vi "DIMPowerSupply.constructor.vi"(0 "name":string, 2 "data in":string, 5 "error in (no error)":errorcluster) -> (14 "i ref out":refnum<vi>, 16 "data out":string, 19 "error out":errorcluster)   [LabVIEW 2014, in "DIMPowerSupply.lvlib"]
doc: "This is the constructor of the DIMPowerSupply class.\n\nauthor: Frank Herfurth, CERN\nmaintainer: Frank Herfurth and Dietrich Beck, GSI\n\nLicense Agreement for this software:\n\nCopyright (C)\nGesellschaft für Schwerionenforschung, GSI\nPlanckstr. 1\n64291 Darmstadt\nGermany\n\nContact: D.Beck@gsi.de \n\nThis program is free software; you can redistribute it and/or modify it under the terms of the \nGNU General Public License as published by the Free Software Foundation; either version 2 of \nthe license, or (at your option) any later version.\n\nThis program is distributed in the hope that it will be useful, but WITHOUT ANY WARRANTY; \nwithout even the implied warranty of MERCHANTABILITY or FITNESS FOR A PARTICULAR PURPOSE. See the GNU General License for more details (http://www.gnu.org).\n\nGesellschaft für Schwerionenforschung, GSI\nPlanckstr. 1, 64291 Darmstadt, Germany\nFor all questions and ideas contact: M.Richter@gsi.de, H.Brand@gsi.de or D.Beck@gsi.de.\nLast update: 16-JUN-2004"
uses:
  DIMPowerSupply.lvlib
  CS_Core/CSApplicationBaseClasses/DeviceBase/DeviceBase.myEventNames.ctl
  CS_Core/CSApplicationBaseClasses/PSChannelBase/PSChannelBase.myEventNames.ctl
  CS_Core/CSSystem/CSSystemLib/CSSystemLib.lvlib
  CSlibraries-extern/DimLVEvent/LVDimInterface/LVDimInterface.lvlib
  CS_Core/CSApplicationBaseClasses/PSChannelBase/PSChannelBase.lvlib
  CS_Core/CSApplicationBaseClasses/DeviceBase/DeviceBase.lvlib
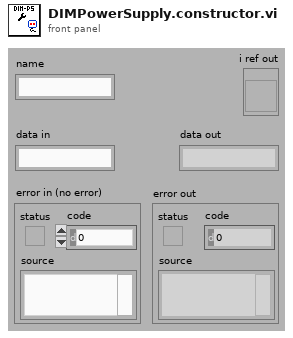
[diagram p1: front panel]
types:
  T1 = enum16{"SetAttribute", "GetAttribute", "CreateAttribute", "DestroyAttribute", "DestroyAllAtributes"}
  T2 = typedef "PSChannelBase.lvlib/PSChannelBase.myEventNames.ctl" = enum16{"lvmsg://EmergencyOff", "lvmsg://SetOnOff", "lvmsg://GetOnOff", "lvmsg://SetVoltage", "lvmsg://GetVoltage", "lvmsg://SetCurrent", "lvmsg://GetCurrent", "lvmsg://SetTripCurrent", "lvmsg://GetTripCurrent", "lvmsg://SetRampUpSpeed", "lvmsg://GetRampUpSpeed", "lvmsg://SetRampDownSpeed", "lvmsg://GetRampDownSpeed", "lvmsg://SetChannelOnOff", "lvmsg://GetChannelOnOff", "lvmsg://SetChannelVoltage", "lvmsg://GetChannelVoltage", "lvmsg://SetChannelCurrent", "lvmsg://GetChannelCurrent", "lvmsg://SetChannelTripCurrent", "lvmsg://GetChannelTripCurrent", "lvmsg://SetChannelRampUpSpeed", "lvmsg://GetChannelRampUpSpeed", "lvmsg://SetChannelRampDownSpeed", "lvmsg://GetChannelRampDownSpeed"}
  T3 = typedef "DeviceBase.lvlib/DeviceBase.myEventNames.ctl" = enum16{"lvmsg://Initialize", "lvmsg://Close", "lvmsg://Configure", "lvmsg://Reset", "lvmsg://IDQuery"}
  T4 = typedef "DIMPowerSupply.lvlib/DIMPowerSupply.i attribute.ctl" = cluster{"ctrlValueID":i32}
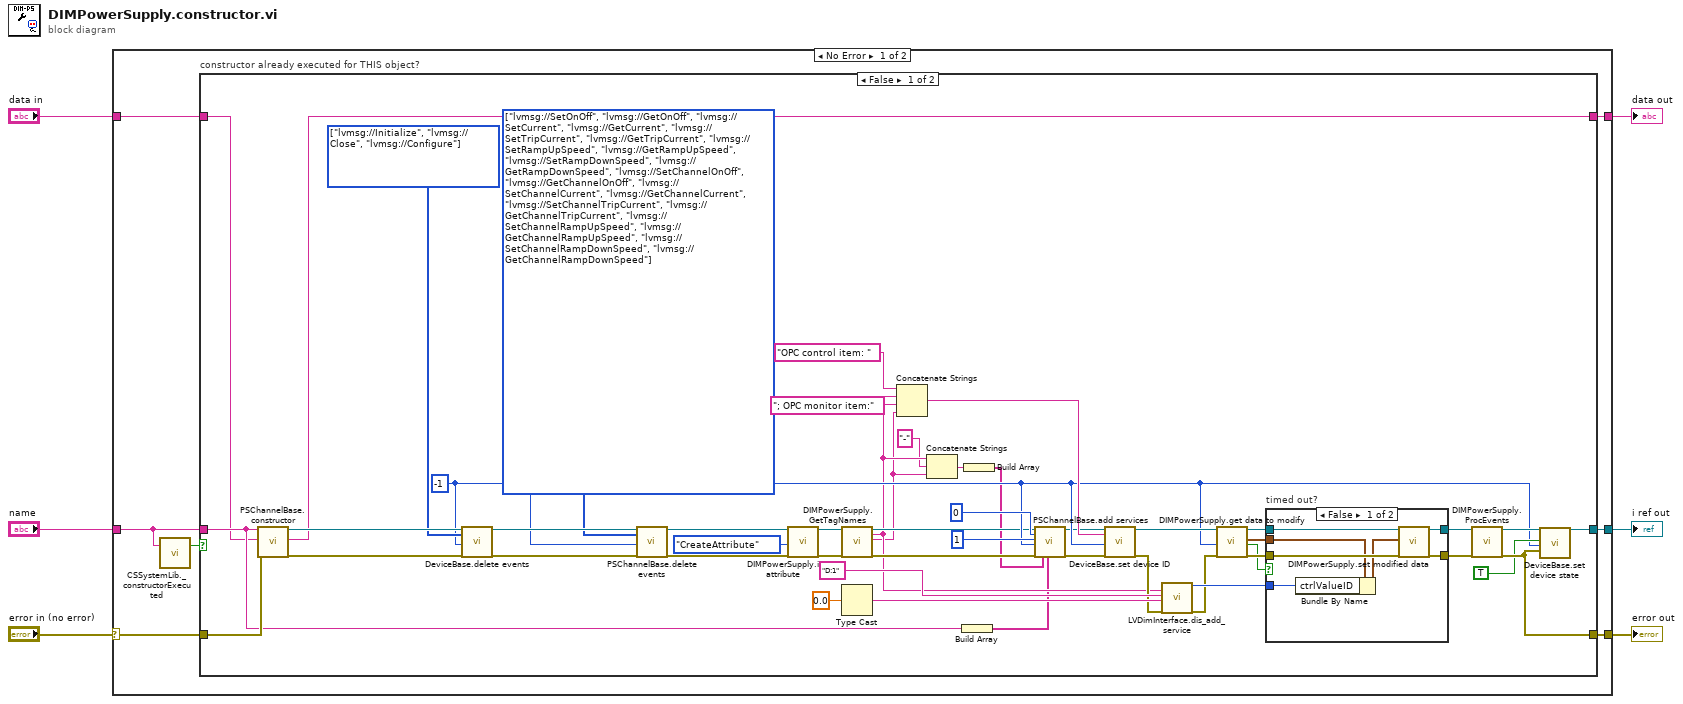
[diagram p0: block diagram]
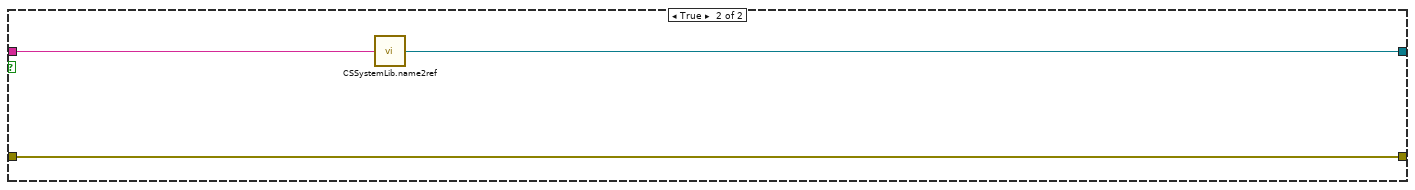
[diagram p3: hidden frame]
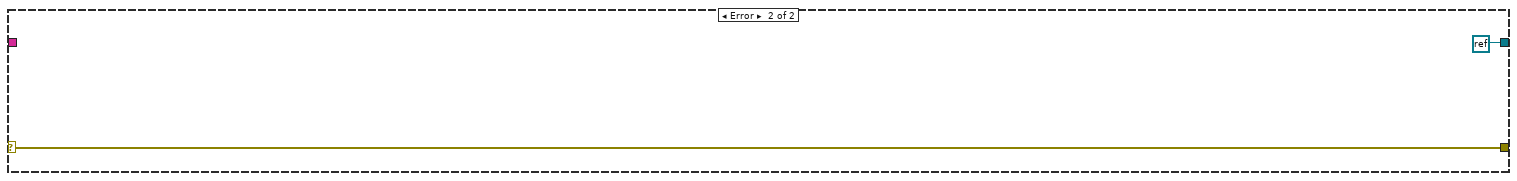
[diagram p4: hidden frame]
diagram:
  n1 = case shown="No Error" "error in (no error)" {
    selector: "error in (no error)" -> [w11 w74]
    tunnel: "name" -> [w10 _]
    tunnel: [w13 refnum<k0> refnum ("Not a Refnum Constant")] -> w5
    tunnel: [w12 w74] -> w4
    tunnel: "data in" -> [w8 _]
    tunnel: [w7 _] -> w1
    frame No Error {
      n2 = call "CSSystemLib._constructorExecuted.vi"("name"=w10) -> ("constructor executed?"=w9:bool)  [unwired: 18 in]
      n3 = case "constructor already executed for THIS object?" shown="False" w9 {
        tunnel: w10 -> [w19 w73]
        tunnel: [w34 w72] -> w13
        tunnel: [w33 w71] -> w12
        tunnel: w11 -> [w60 w71]
        tunnel: w8 -> [w15 _]
        tunnel: [w14 _] -> w7
        frame False {
          w41 = T2[] [enum."lvmsg://SetOnOff", enum."lvmsg://GetOnOff", enum."lvmsg://SetCurrent", enum."lvmsg://GetCurrent", enum."lvmsg://SetTripCurrent", enum."lvmsg://GetTripCurrent", enum."lvmsg://SetRampUpSpeed", enum."lvmsg://GetRampUpSpeed", enum."lvmsg://SetRampDownSpeed", enum."lvmsg://GetRampDownSpeed", enum."lvmsg://SetChannelOnOff", enum."lvmsg://GetChannelOnOff", enum."lvmsg://SetChannelCurrent", enum."lvmsg://GetChannelCurrent", enum."lvmsg://SetChannelTripCurrent", enum."lvmsg://GetChannelTripCurrent", enum."lvmsg://SetChannelRampUpSpeed", enum."lvmsg://GetChannelRampUpSpeed", enum."lvmsg://SetChannelRampDownSpeed", enum."lvmsg://GetChannelRampDownSpeed"] items=["lvmsg://EmergencyOff", "lvmsg://SetOnOff", "lvmsg://GetOnOff", "lvmsg://SetVoltage", "lvmsg://GetVoltage", "lvmsg://SetCurrent", "lvmsg://GetCurrent", "lvmsg://SetTripCurrent", "lvmsg://GetTripCurrent", "lvmsg://SetRampUpSpeed", "lvmsg://GetRampUpSpeed", "lvmsg://SetRampDownSpeed", "lvmsg://GetRampDownSpeed", "lvmsg://SetChannelOnOff", "lvmsg://GetChannelOnOff", "lvmsg://SetChannelVoltage", "lvmsg://GetChannelVoltage", "lvmsg://SetChannelCurrent", "lvmsg://GetChannelCurrent", "lvmsg://SetChannelTripCurrent", "lvmsg://GetChannelTripCurrent", "lvmsg://SetChannelRampUpSpeed", "lvmsg://GetChannelRampUpSpeed", "lvmsg://SetChannelRampDownSpeed", "lvmsg://GetChannelRampDownSpeed"] ("events")
          w42 = T3[] [enum."lvmsg://Initialize", enum."lvmsg://Close", enum."lvmsg://Configure"] items=["lvmsg://Initialize", "lvmsg://Close", "lvmsg://Configure", "lvmsg://Reset", "lvmsg://IDQuery"] ("events")
          w29 = -1 ("ms timeout (10000)")
          n4 = call "PSChannelBase.constructor.vi"("name"=w19, "data in"=w15, "error in (no error)"=w60) -> ("i ref out"=w46:refnum<vi>, "data out"=w14:string, "error out"=w45:errorcluster)  [unwired: 14 in]
          n5 = call "DeviceBase.delete events.vi"("i ref in"=w46, "events"=w42, "ms timeout (10000)"=w29, "error in (no error)"=w45) -> ("i ref out"=w44:refnum<vi>, "error out"=w43:errorcluster)  [unwired: 13 in, 1 out]
          n6 = call "PSChannelBase.delete events.vi"("i ref in"=w44, "events"=w41, "ms timeout (10000)"=w29, "error in (no error)"=w43) -> ("i ref out"=w17:refnum<vi>, "error out"=w16:errorcluster)  [unwired: 13 in, 1 out]
          n7 = call "DIMPowerSupply.i attribute.vi"("VI Refnum"=w17, "Action"=T1."CreateAttribute", "error in (no error)"=w16) -> ("VI Refnum out"=w51:refnum<vi>, "error out"=w47:errorcluster)  [unwired: 14 in, 1 out]
          n8 = call "DIMPowerSupply.GetTagNames.vi"("i ref in"=w51, "error in (no error)"=w47) -> ("i ref out"=w28:refnum<vi>, "CtrTagName"=w24:string, "MonTagName"=w22:string, "error out"=w27:errorcluster)  [unwired: 14 in]
          n9 = Type Cast(x=0.0) -> (*(type *) &x=w53:string)  [unwired: 1 in]
          n10 = Concatenate Strings("OPC control item: " ("string"), w24, "; OPC monitor item:" ("string"), w22) -> (w37:string)
          n11 = Concatenate Strings(w24, "-" ("string"), w22) -> (w21:string)
          n12 = Build Array(w19) -> (w18:string[])
          n13 = Build Array(w21) -> (w20:string[])
          n14 = call "PSChannelBase.add services.vi"("i ref in"=w28, "defaultChannelIndex"=0, "nofChannels"=1, "ms timeout (10000)"=w29, "error in (no error)"=w27, "physicalNames"=w20, "logicalNames"=w18) -> ("i ref out"=w25:refnum<vi>, "error out"=w26:errorcluster)  [unwired: 10 in, 1 out]
          n15 = call "DeviceBase.set device ID.vi"("i ref in"=w25, "deviceID"=w37, "ms timeout (10000)"=w29, "error in (no error)"=w26) -> ("i ref out"=w36:refnum<vi>, "error out"=w38:errorcluster)  [unwired: 13 in, 1 out]
          n16 = call "LVDimInterface.dis_add_service.vi"("serviceName"=w24, "typeDescriptor"="D:1", "data"=w53, "error in (no error)"=w38) -> ("my_serviceID"=w52:i32, "error out"=w48:errorcluster)  [unwired: 14 in]
          n17 = call "DIMPowerSupply.get data to modify.vi"("i ref in"=w36, "ms timeout (10000)"=w29, "error in (no error)"=w48) -> ("i ref out"=w58:refnum<vi>, "i attribute"=w55:T4, "timed out"=w56:bool, "error out"=w57:errorcluster)  [unwired: 13 in]
          n18 = case "timed out?" shown="False" w56 {
            tunnel: [w68 w70] -> w50
            tunnel: w58 -> [w67 w70]
            tunnel: [w65 w69] -> w49
            tunnel: w57 -> [w66 w69]
            tunnel: w55 -> [w64 _]
            tunnel: w52 -> [w62 _]
            frame False {
              n19 = Bundle By Name(cluster=w64, "ctrlValueID"=w62) -> (w63:T4)
              n20 = call "DIMPowerSupply.set modified data.vi"("i ref in"=w67, "i attribute"=w63, "error in (no error)"=w66) -> ("i ref out"=w68:refnum<vi>, "error out"=w65:errorcluster)  [unwired: 15 in]
            }
            frame True {
            }
          }
          n21 = call "DIMPowerSupply.ProcEvents.vi"("i ref in"=w50, "error in (no error)"=w49) -> ("i ref out"=w35:refnum<vi>, "error out"=w33:errorcluster)  [unwired: 16 in]
          n22 = call "DeviceBase.set device state.vi"("i ref in"=w35, "implicit"=TRUE, "ms timeout (10000)"=w29, "device error"=w33) -> ("i ref out"=w34:refnum<vi>)  [unwired: 13 in, 2 out]
        }
        frame True {
          n23 = call "CSSystemLib.name2ref.vi"("name"=w73) -> ("obj refnum"=w72:refnum<vi>)
        }
      }
    }
    frame Error {
    }
  }
  "i ref out" <- w5
  "error out" <- w4
  "data out" <- w1
